vi "EventLog.ListFiles.vi"(7 "Sets in":T5 caption="Event.Sets" {"Source" items=["0", "1", "2", "3", "4", "5", "6", "7"]; "dtm_End" format="%<%.1X\n%x>T"; "dtm_Begin" format="%<%.1X\n%x>T"}, 8 "error in":errorcluster, 9 "Size":i32=50, 11 "Path":path) -> (0 "error out":errorcluster, 2 "Events":T1[](array[typedef]) {"ts" format="%<%X\n%x>T"}, 5 "Sets out":T5 {"dtm_End" format="%<%.1X\n%x>T"; "dtm_Begin" format="%<%.1X\n%x>T"})   [LabVIEW 2016]
uses:
  EventLog.Gui.Sets.ctl
  EventLog.EventLevelOperatorGui.ctl
  EventLog.EventGui.ctl
  EventLog.EventLevel.ctl
  EventLog.EventSource.ctl
  Translator/Translator.Message.ctl
  EventLog.Buffer.Action.ctl
panel:
  out "reversed array":T1[](array[typedef]) {"ts" format="%<%X\n%x>T"}
  out "percentage":dbl format="%#.2f"
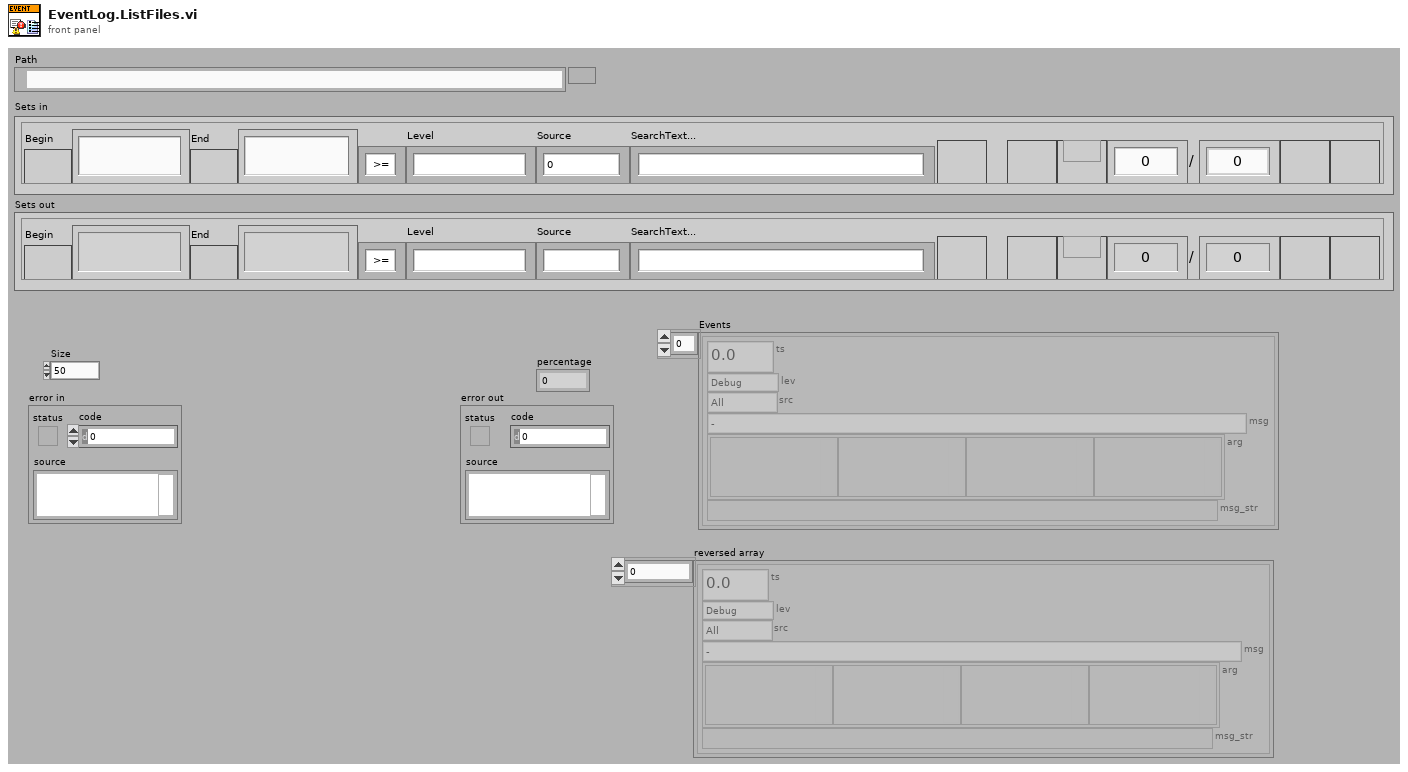
[diagram p1: front panel]
types:
  T1 = typedef "EventLog.EventGui.ctl" = cluster{"ts":dbl, "lev":T2, "src":T3, "msg":T4, "arg":variant[], "msg_str":string}
  T2 = typedef "EventLog.EventLevel.ctl" = enum8{"Debug", "Info", "Warning", "Error"}
  T3 = typedef "EventLog.EventSource.ctl" = enum16{"All", "Gui", "Cache", "PLC1", "PLC2", "PLC3", "DB", "DB01", "DB02", "DB03", "DB04", "DB05", "DB06", "DB07", "DB08", "DB09", "DB10", "DB11", "DB12", "DB13", "DB14", "DB15", "DB16"}
  T4 = typedef "Translator.Message.ctl" = enum16{"-", "Event confirmed", "Log out", "Log in", "Shutdown", "Cancel", "Start", "Continue", "Stop", "On", "Off", "OK", "NOK", "NOK %s", "This", "Prev", "Home", "Work", "In progress...", "Missing", "Empty", "Hardware failure", "Initial", "Error %d >> %s", "Error %d >> %s >> %s", "Starting %s", "Quitting %s", "Configured", "Initializing", "Quitting", "Loading", "Running %s", "Stopped", "Summary", "Do you want to continue?", "Do you want to exit?", "Log out?", "System", "All", "IDLE", "Translating...%s", "Not found", "Alarm %s", "Run", "Skip", "Abort", "Repeat", "Please wait...", "Database disconnected", "Login to database successful", "Login to database failed: %d; %s", "Get process step data for %s", "Changeover off", "Changeover into %s", "Product %s | %s found in cache with status %d at previous station", "Product %s | %s found in database with status %d at previous station", "Product %s | %s not found in cache at previous station", "Product %s | %s not found in database at previous station", "Product %s | %s found in cache with status %d at this station (%d repetion)", "Product %s | %s found in database with status %d at this station (%d repetition)", "Product %s | %s not found in cache at this station", "Product %s | %s not found in database at this station", "Product %s | %s found in cache for component %s | %s", "Product %s | %s found in database for component %s | %s", "Product not found in cache for component %s | %s", "Product not found in database for component %s | %s", "Product %s | %s connected with component %s | %s (cache)", "Product %s | %s connected with component %s | %s (database)", "New data for %s | %s (cache)", "New data for %s | %s (database)", "File %s moved (cache)", "File %s deleted (cache)", "Msg %d >> %s", "PLC LifeBit Failure", "Reconnecting DB", "Reconnecting PLC", "Free disk space is below 1GB - contact technician", "Unable to check product status", "Product %s SN %s checked in DB"}
  T5 = typedef "EventLog.Gui.Sets.ctl" = cluster{"IncludeBegin":bool, "dtm_Begin":timestamp, "IncludeEnd":bool, "dtm_End":timestamp, "Events Level Operator":T6, "Level":u16, "Source":u16, "SearchText":string, "Refresh":bool, "Pages":i32, "PageNo":i32, "First":bool, "Prev":bool, "Next":bool, "Last":bool}
  T6 = typedef "EventLog.EventLevelOperatorGui.ctl" = enum16{">=", "=", "<="}
  T7 = typedef "EventLog.Buffer.Action.ctl" = enum16{"init", "re-init", "clear", "set translator", "translate", "add", "get"}
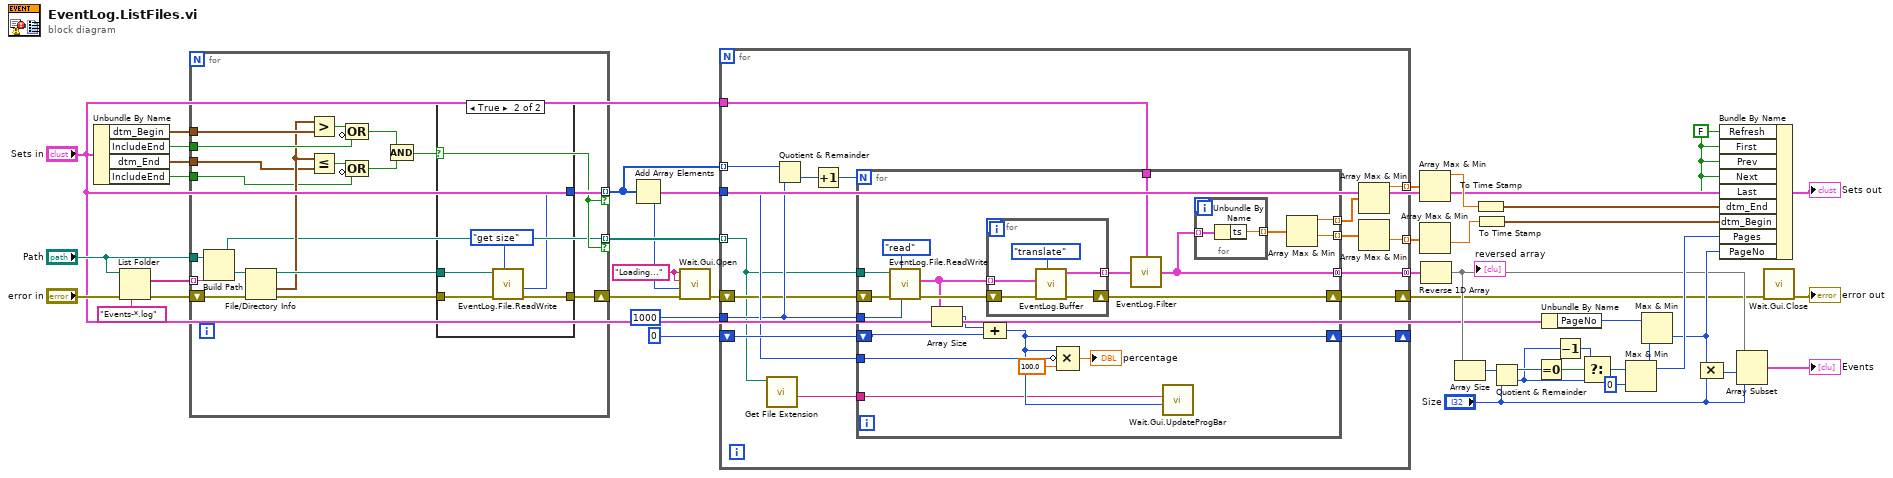
[diagram p0: block diagram]
diagram:
  w1 = "Loading..." ("Status (\"\")")
  w7 = FALSE ("Refresh")
  n1 = Unbundle By Name("Sets in") -> ("dtm_Begin"=w39:timestamp, "IncludeEnd"=w38:bool, "dtm_End"=w37:timestamp, "IncludeEnd"=w36:bool)
  n2 = List Folder(path="Path", pattern="Events-*.log", error in="error in") -> (filenames=w42:string[], error out=w41:errorcluster)  [unwired: 1 in, 2 out]
  n3 = for {
    tunnel: "Path" -> [w61]
    tunnel: w42 -> [w60] mode=indexing
    shift-right: [w59] -> w6
    shift-left: w41 -> [w58]
    tunnel: [w44] -> w32 mode=indexing if=w45
    tunnel: w39 -> [w54]
    tunnel: w38 -> [w53]
    tunnel: w37 -> [w50]
    tunnel: w36 -> [w49]
    tunnel: [w46] -> w31 mode=indexing if=w45
    n4 = Build Path(base path=w61, name or relative path=w60) -> (appended path=w44:path)
    n5 = File/Directory Info(path=w44, error in=w58) -> (path out=w57:path, last mod=w51:timestamp, error out=w56:errorcluster)  [unwired: 4 out]
    n6 = Greater?(x=w51, y=w54) -> (0:w55:bool)
    n7 = Less Or Equal?(x=w51, y=w50) -> (x <= y?=w52:bool)
    n8 = Compound Arithmetic op=OR(w55, invert w53) -> (w48:bool)
    n9 = Compound Arithmetic op=OR(w52, invert w49) -> (w47:bool)
    n10 = Compound Arithmetic op=AND(w48, w47) -> (w45:bool)
    n11 = case shown="True" w45 {
      tunnel: [w62 w64] -> w59
      tunnel: w57 -> [_ w66]
      tunnel: w56 -> [w62 w65]
      tunnel: [_ w63] -> w46
      frame False {
      }
      frame True {
        n12 = call "EventLog.File.ReadWrite.vi"("action (read)"=enum16{"read", "write", "get size"}."get size", "error in"=w65, "file"=w66) -> ("error out"=w64:errorcluster, "offset [B]"=w63:i64)  [unwired: 4 in, 3 out]
      }
    }
  }
  n13 = Add Array Elements(numeric array=w31) -> (sum=w4:i64)
  n14 = call "Wait.Gui.Open.vi"("error in (no error)"=w6, "ProgBarSize (0)"=w4, "Status (\"\")"=w1, "Msg"=w1) -> ("error out"=w5:errorcluster)  [unwired: 7 in]
  n15 = for {
    tunnel: w4 -> [w82]
    tunnel: i64 1000 ("y") -> [w81]
    tunnel: w32 -> [w70] mode=indexing
    tunnel: w31 -> [w79] mode=indexing
    tunnel: "Sets in" -> [w78]
    shift-right: [w77] -> _
    shift-left: 0 -> [w83]
    tunnel: [w76] -> w30 mode=indexing
    tunnel: [w75] -> w29 mode=indexing
    shift-right: [w74] -> w3
    shift-left: w5 -> [w80]
    tunnel: [w71] -> w14 mode=concatenating
    n16 = call <vilib>:"Get File Extension.vi"("file"=w70) -> ("filename without extension"=w69:string)  [unwired: 6 in, 4 out]
    n17 = Quotient & Remainder(x=w79, y=w81) -> (floor(x/y)=w84:i64)  [unwired: 1 out]
    n18 = Increment(x=w84) -> (x+1=w68:i64)
    n19 = for {
      N: w68 -> [_]
      shift-right: [w101] -> w74
      shift-left: w80 -> [w103]
      shift-right: [w86] -> w77
      shift-left: w83 -> [w99]
      tunnel: w82 -> [w98]
      tunnel: w81 -> [w97]
      tunnel: w70 -> [w92]
      tunnel: w78 -> [w91]
      tunnel: [w89] -> w72 mode=indexing
      tunnel: [w88] -> w73 mode=indexing
      tunnel: [w87] -> w71 mode=concatenating
      tunnel: w69 -> [w85]
      n20 = call "EventLog.File.ReadWrite.vi"("read count (ALL)"=w97, "action (read)"=enum16{"read", "write", "get size"}."read", "error in"=w103, "file"=w92) -> ("error out"=w102:errorcluster, "Events out"=w94:T1[])  [unwired: 3 in, 3 out]
      n21 = Array Size(array=w94) -> (size(s)=w93:i32)
      n22 = Compound Arithmetic op=ADD(w93, w99) -> (w86:i32)
      n23 = for {
        tunnel: w94 -> [w111] mode=indexing
        shift-right: [w109] -> w101
        shift-left: w102 -> [w110]
        tunnel: [w107] -> w100 mode=indexing
        n24 = call "EventLog.Buffer.vi"("action (get)"=EventLog.Buffer.Action."translate" ("action (read)"), "error in"=w110, "Event in"=w111) -> ("error out"=w109:errorcluster, "Event out"=w107:T1)  [unwired: 5 in, 2 out]
      }
      n25 = Compound Arithmetic op=MULTIPLY(w86, invert w98, 100.0 ("y")) -> (→"percentage":dbl)
      n26 = call "EventLog.Filter.vi"("data in"=w100, "Event.Sets"=w91) -> ("data out"=w87:T1[])
      n27 = call "Wait.Gui.UpdateProgBar.vi"("ProgBar (0)"=w86, "status (\"\")"=w85) -> ()  [unwired: 9 in, 1 out]
      n28 = for {
        tunnel: w87 -> [w106] mode=indexing
        tunnel: [w105] -> w90 mode=indexing
        n29 = Unbundle By Name(w106) -> ("ts"=w105:dbl)
      }
      n30 = Array Max & Min(array=w90) -> (max value=w89:dbl, min value=w88:dbl)  [unwired: 2 out]
    }
    n31 = Array Max & Min(array=w72) -> (max value=w76:dbl)  [unwired: 3 out]
    n32 = Array Max & Min(array=w73) -> (min value=w75:dbl)  [unwired: 3 out]
  }
  n33 = Array Max & Min(array=w30) -> (max value=w28:dbl)  [unwired: 3 out]
  n34 = Array Max & Min(array=w29) -> (min value=w27:dbl)  [unwired: 3 out]
  n35 = Reverse 1D Array(array=w14) -> (reversed array=w9:T1[])
  "reversed array" <- w9
  n36 = Array Size(array=w9) -> (size(s)=w11:i32)
  n37 = To Time Stamp(1:w28) -> (0:w26:timestamp)
  n38 = To Time Stamp(1:w27) -> (0:w25:timestamp)
  n39 = Quotient & Remainder(x=w11, y="Size") -> (x-y*floor(x/y)=w22:i32, floor(x/y)=w20:i32)
  n40 = Equal To 0?(x=w22) -> (x = 0?=w21:bool)
  n41 = Unbundle By Name("Sets in") -> ("PageNo"=w16:i32)
  n42 = Decrement(x=w20) -> (x-1=w19:i32)
  n43 = Select(t=w19, s=w21, f=w20) -> (s? t:f=w18:i32)
  n44 = Max & Min(x=w18, y=0) -> (max(x,y)=w13:i32)  [unwired: 1 out]
  n45 = Max & Min(x=w16, y=w13) -> (min(x,y)=w12:i32)  [unwired: 1 out]
  n46 = Compound Arithmetic op=MULTIPLY(w12, "Size") -> (w15:i32)
  n47 = Bundle By Name(cluster="Sets in", "Refresh"=w7, "First"=w7, "Prev"=w7, "Next"=w7, "Last"=w7, "dtm_End"=w26, "dtm_Begin"=w25, "Pages"=w13, "PageNo"=w12) -> (→"Sets out":T5)
  n48 = Array Subset(array=w9, index=w15, length="Size") -> (→"Events":T1[])
  n49 = call "Wait.Gui.Close.vi"("error in (no error)"=w3) -> ("error out"=→"error out":errorcluster)  [unwired: 10 in]
